vi "test interpolate.vi"() -> ()   [LabVIEW 2016]
uses:
  <vilib>/Analysis/1siggen.llb/Ramp Pattern by Delta.vi
  <vilib>/gmath/NI_Gmath.lvlib
  <vilib>/Analysis/NI_AALBase.lvlib
panel:
  out "1D Interpolation Graph":cluster{"xi used":dbl[], "yi":dbl[]}(graph)
  in  "method":i32(ring)=1 items=["nearest", "linear", "spline", "cubic Hermite", "Lagrange"]
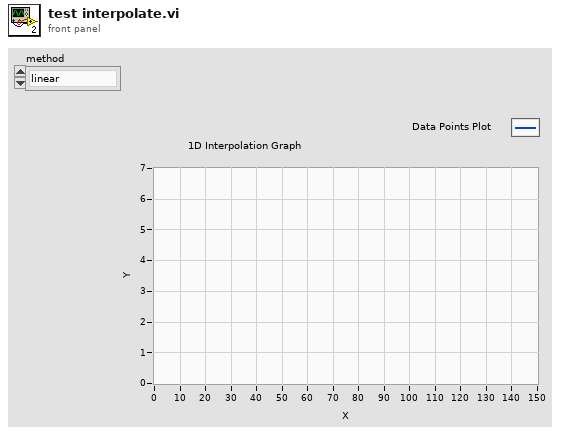
[diagram p1: front panel]
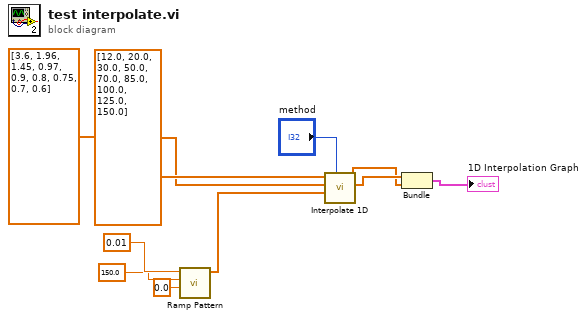
[diagram p0: block diagram]
diagram:
  n1 = call-poly <vilib>:"Ramp Pattern.vi"("start"=0.0, "end"=150.0, "delta"=0.01) -> ("Ramp Pattern"=w4:dbl[])  [unwired: 6 in, 2 out]
  n2 = call <vilib>:"Interpolate 1D.vi"("method"="method", "xi"=w4, "X"=dbl[] [12.0, 20.0, 30.0, 50.0, 70.0, 85.0, 100.0, 125.0, 150.0], "Y"=dbl[] [3.6, 1.96, 1.45, 0.97, 0.9, 0.8, 0.75, 0.7, 0.6]) -> ("xi used"=w3:dbl[], "yi"=w2:dbl[])  [unwired: 5 in, 1 out]
  n3 = Bundle("xi used"=w3, "yi"=w2) -> (→"1D Interpolation Graph":cluster{"xi used":dbl[], "yi":dbl[]})  [unwired: 1 in]
